vi "Constrained Nonlinear Optimization.vi"(0 "start":dbl[](array[numeric]), 1 "objective and constraint function":T3, 2 "function data":T2, 5 "bounds":T5, 9 "beginning state":T1, 11 "error in (no error)":errorcluster, 12 "cno settings":T6={"constraint weight"=1.0, "maximum minor iterations"=10}, 13 "stopping criteria":T4={"function tolerance"=1e-06, "parameter tolerance"=1e-06, "max iterations"=100, "max function calls"=1000, "gradient tolerance"=1e-06, "max time (sec)"=-1.0}) -> (3 "number of function calls":i32, 4 "minimum":dbl[](array[numeric]), 6 "f(minimum)":dbl, 10 "ending state":T1, 15 "error out":errorcluster)   [LabVIEW 2020, in "NI_Gmath.lvlib"]
doc: "Solves a general nonlinear optimization problem with nonlinear equality constraint and nonlinear inequality constraint bounds using a sequential quadratic programming method."
uses:
  NI_Gmath.lvlib
  cno_tuning parameters.ctl
  cno_bounds.ctl
  cno_initial values.ctl
  stopping criteria.ctl
  cno_user objective function ref.ctl
  objective function data.ctl
  NI_AALPro.lvlib
panel:
  in  "ending state 2":T1
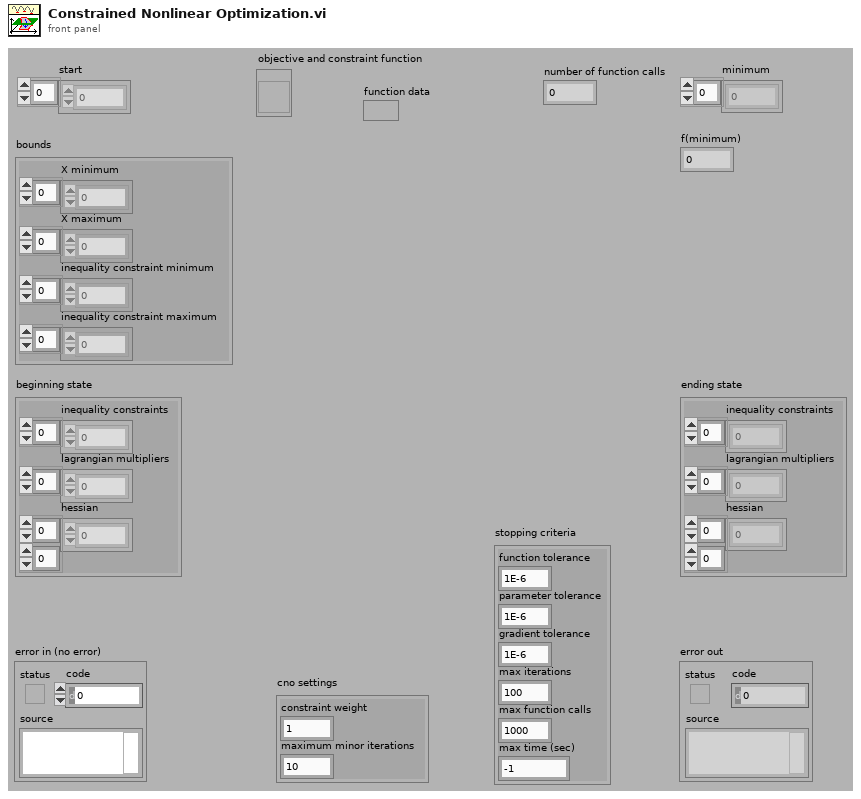
[diagram p1: front panel]
types:
  T1 = typedef "NI_Gmath.lvlib/cno_initial values.ctl" = cluster{"inequality constraints":dbl[], "lagrangian multipliers":dbl[], "hessian":dbl[][]}
  T2 = typedef "NI_Gmath.lvlib/objective function data.ctl" = variant
  T3 = typedef "NI_Gmath.lvlib/cno_user objective function ref.ctl" = refnum<vi>
  T4 = typedef "NI_Gmath.lvlib/stopping criteria.ctl" = cluster{"function tolerance":dbl, "parameter tolerance":dbl, "max iterations":i32, "max function calls":i32, "gradient tolerance":dbl, "max time (sec)":dbl}
  T5 = typedef "NI_Gmath.lvlib/cno_bounds.ctl" = cluster{"X minimum":dbl[], "X maximum":dbl[], "inequality constraint minimum":dbl[], "inequality constraint maximum":dbl[]}
  T6 = typedef "NI_Gmath.lvlib/cno_tuning parameters.ctl" = cluster{"constraint weight":dbl, "maximum minor iterations":i32}
  T7 = cluster{"objective and constraint function":T3, "function data":T2}
  T8 = typedef "NI_Gmath.lvlib/stopping criteria with time.ctl" = cluster{"function tolerance":dbl, "parameter tolerance":dbl, "max iterations":i32, "max function calls":i32, "gradient tolerance":dbl, "max time (sec)":dbl, "initial tick count":u32}
  T9 = typedef "NI_Gmath.lvlib/cno_data.ctl" = cluster{"NP":i32, "NIC":i32, "NEC":i32, "NC":i32, "NPIC":i32, "parameterBounds":bool, "alpha1":dbl, "alpha2":dbl, "alpha3":dbl, "alpha4":dbl, "CH":i32, "MM":i32, "tolerance":dbl}
  T10 = enum32{"Identity", "Diagonal", "Toepliz", "Vandermonde", "Companion"}
  T11 = typedef "NI_Matrix.lvlib/RealMatrix.ctl" = dbl[][]
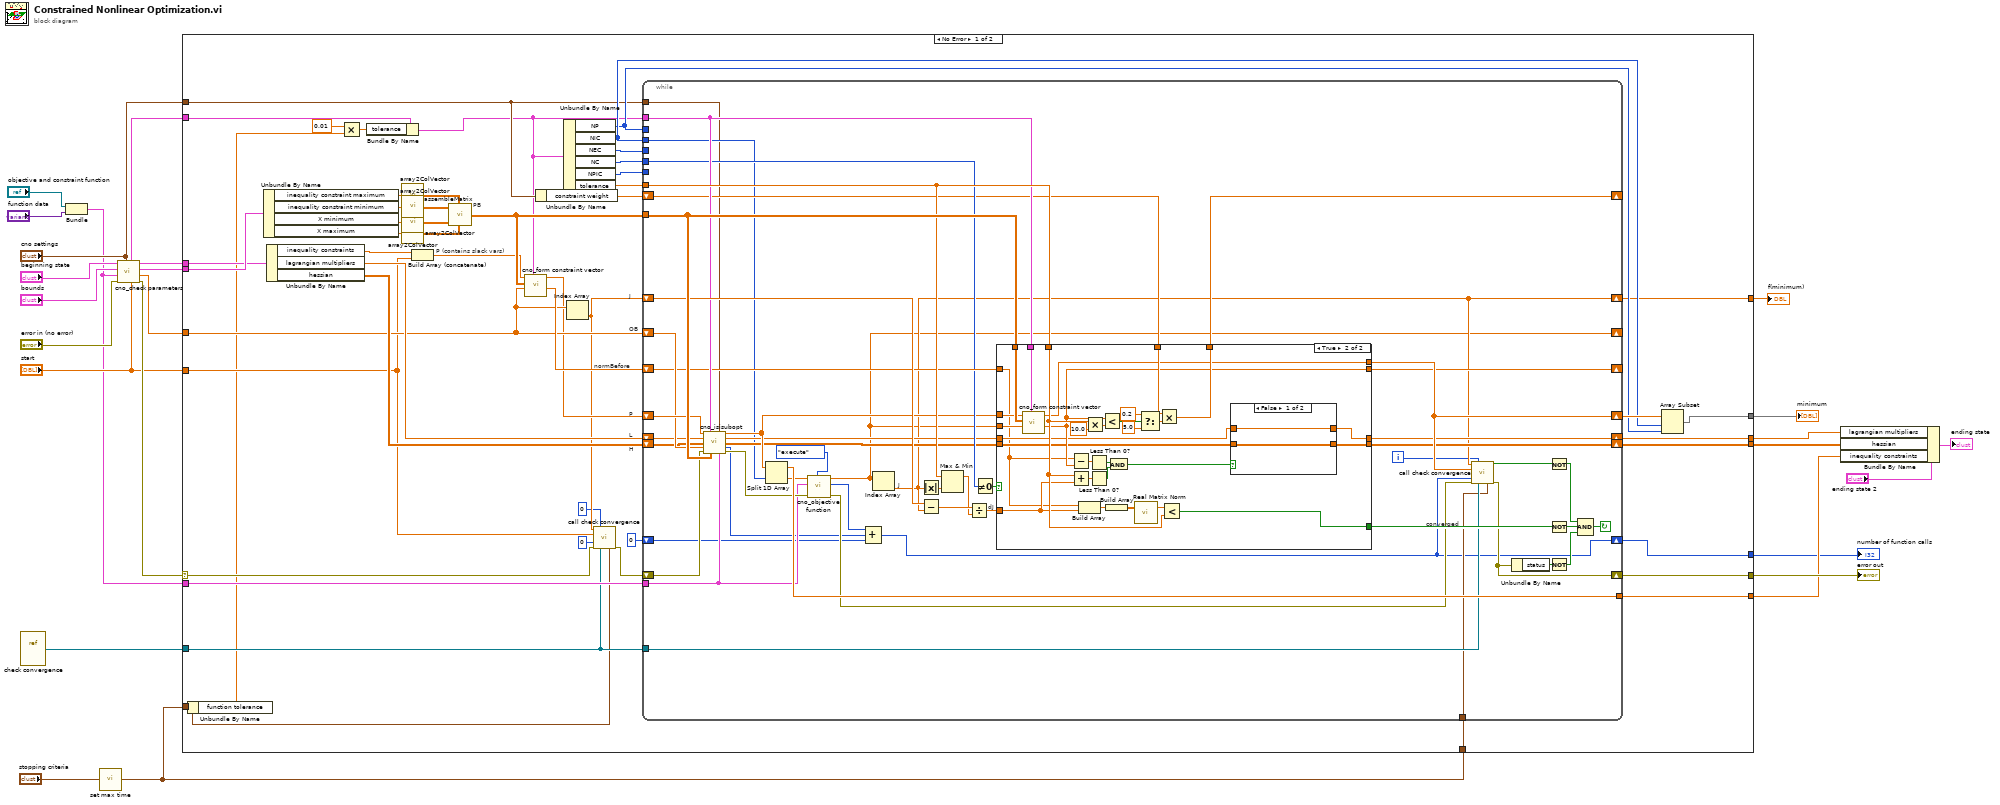
[diagram p0: block diagram]
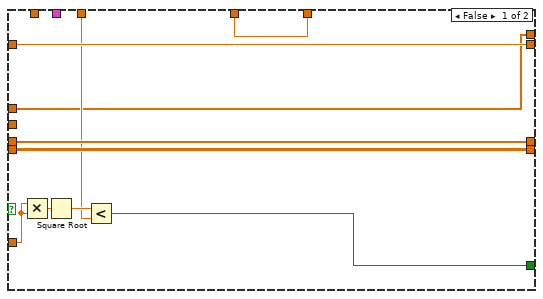
[diagram p2: hidden frame]
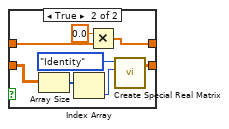
[diagram p3: hidden frame]
diagram:
  n1 = vi-ref "check convergence.vi"() -> ("vi reference"=w7:refnum<vi>)
  n2 = Bundle("objective and constraint function"="objective and constraint function", "function data"="function data") -> (w4:T7)  [unwired: 1 in]
  n3 = call "set max time.vi"("stopping criteria"="stopping criteria") -> ("stopping criteria"=w2:T8)
  n4 = call "cno_check parameters.vi"("initial parameters"="start", "tuning parameters"="cno settings", "error in (no error)"="error in (no error)", "user defined functions"=w4, "limits"="bounds", "state values"="beginning state") -> ("error out"=w19:errorcluster, "OB0"=w18:dbl[], "limits out"=w21:T5, "state values out"=w20:T1, "cno data"=w17:T9)  [unwired: 1 in]
  n5 = case shown="No Error" w19 {
    selector: w19 -> [w41 w176]
    tunnel: w4 -> [w58 _]
    tunnel: w20 -> [w74 _]
    tunnel: w21 -> [w75 _]
    tunnel: w18 -> [w56 _]
    tunnel: "cno settings" -> [w31 _]
    tunnel: w17 -> [w30 _]
    tunnel: [w55 w176] -> w16
    tunnel: [w49 _] -> w10
    tunnel: [w54 _] -> w13
    tunnel: [w53 _] -> w12
    tunnel: [w45 _] -> w15
    tunnel: [w52 _] -> w14
    tunnel: "start" -> [w43 _]
    tunnel: [w27 _] -> w8
    tunnel: w7 -> [w39 _]
    tunnel: w2 -> [w38 _]
    tunnel: w2 -> [w34 _]
    frame No Error {
      # "OB"
      # "H"
      # "L"
      # "P"
      # "normBefore"
      # "J"
      # "PB"
      # "P (contains slack vars)"
      n6 = Unbundle By Name(w34) -> ("function tolerance"=w33:dbl)
      n7 = Unbundle By Name(w75) -> ("inequality constraint maximum"=w44:dbl[], "inequality constraint minimum"=w70:dbl[], "X minimum"=w72:dbl[], "X maximum"=w71:dbl[])
      n8 = Unbundle By Name(w74) -> ("inequality constraints"=w73:dbl[], "lagrangian multipliers"=w62:dbl[], "hessian"=w61:dbl[][])
      n9 = Multiply(x=0.01, y=w33) -> (x*y=w32:dbl)
      n10 = Bundle By Name(cluster=w30, "tolerance"=w32) -> (w29:T9)
      n11 = call "array2ColVector.vi"("vector"=w44) -> ("col vector"=w66:dbl[][])
      n12 = call "array2ColVector.vi"("vector"=w70) -> ("col vector"=w67:dbl[][])
      n13 = call "array2ColVector.vi"("vector"=w72) -> ("col vector"=w69:dbl[][])
      n14 = call "array2ColVector.vi"("vector"=w71) -> ("col vector"=w68:dbl[][])
      n15 = Build Array (concatenate)(w73, w43) -> (w63:dbl[])
      n16 = call "assembleMatrix.vi"("A"=w67, "B"=w66, "C"=w69, "D"=w68) -> ("ABCD"=w65:dbl[][])  [unwired: 1 in]
      n17 = call "cno_form constraint vector.vi"("cno data"=w29, "OB"=w56, "PB"=w65, "P in"=w63) -> ("norm"=w64:dbl, "P out"=w51:dbl[])  [unwired: 6 in]
      n18 = Unbundle By Name(w31) -> ("constraint weight"=w57:dbl)
      n19 = Unbundle By Name(w29) -> ("NP"=w47:i32, "NIC"=w48:i32, "NEC"=w46:i32, "NC"=w60:i32, "NPIC"=w59:i32, "tolerance"=w28:dbl)
      n20 = Index Array(array=w56) -> (element=w42:dbl)  [unwired: 1 in]
      n21 = call "call check convergence.vi"("f"=w42, "current iteration"=0, "X"=w43, "number of function evaluations"=0, "error in"=w41, "vi reference"=w39, "stopping criteria"=w34) -> ("error out"=w40:errorcluster)  [unwired: 4 in, 4 out]
      n22 = while {
        tunnel: w65 -> [w124]
        shift-right: [w113] -> _
        shift-left: w64 -> [w109]
        tunnel: w31 -> [w86]
        shift-right: [w112] -> w52
        shift-left: w62 -> [w97]
        shift-right: [w111] -> w54
        shift-left: w61 -> [w99]
        shift-right: [w125] -> w50
        shift-left: w51 -> [w122]
        tunnel: w29 -> [w116]
        tunnel: w47 -> [_]
        tunnel: w48 -> [w95]
        tunnel: w46 -> [_]
        tunnel: w60 -> [w103]
        tunnel: w59 -> [_]
        shift-right: [w91] -> w55
        shift-left: w40 -> [w121]
        tunnel: w58 -> [w80]
        shift-right: [w94] -> w45
        shift-left: w42 -> [w120]
        tunnel: w28 -> [w123]
        shift-right: [w114] -> _
        shift-left: w57 -> [w100]
        shift-right: [w83] -> _
        shift-left: w56 -> [w115]
        tunnel: [w101] -> w53
        tunnel: w39 -> [w92]
        tunnel: w38 -> [w87]
        shift-right: [w76] -> w27
        shift-left: 0 -> [w78]
        i -> [w93]
        stop <- w88 continue-if-true
        # "J"
        # "converged"
        # "dJ"
        n23 = call "cno_isisubopt.vi"("P"=w122, "cno data"=w116, "tuning parameters"=w86, "L"=w97, "H"=w99, "OB"=w115, "error in (no error)"=w121, "PB"=w124, "user defined functions"=w80) -> ("P"=w102:dbl[], "L"=w96:dbl[], "H"=w98:dbl[][], "number of function calls"=w79:i32, "error out"=w82:errorcluster)  [unwired: 2 in]
        n24 = Split 1D Array(array=w102, index=w95) -> (first subarray=w101:dbl[], second subarray=w84:dbl[])
        n25 = call "cno_objective function.vi"("function"=enum16{"initialize", "execute"}."execute", "error in (no error)"=w82, "user defined functions"=w80, "X"=w84) -> ("error out"=w81:errorcluster, "num function calls"=w77:i32, "F(X)"=w83:dbl[])  [unwired: 5 in]
        n26 = Compound Arithmetic op=ADD(w77, w79, w78) -> (w76:i32)
        n27 = Index Array(array=w83) -> (element=w94:dbl)  [unwired: 1 in]
        n28 = Absolute Value(x=w94) -> (abs(x)=w119:dbl)
        n29 = Subtract(x=w120, y=w94) -> (x-y=w118:dbl)
        n30 = Max & Min(x=w123, y=w119) -> (max(x,y)=w117:dbl)  [unwired: 1 out]
        n31 = Divide(x=w118, y=w117) -> (x/y=w110:dbl)
        n32 = Not Equal To 0?(x=w103) -> (x != 0?=w104:bool)
        n33 = case shown="True" w104 {
          tunnel: w123 -> [w128 w165]
          tunnel: w124 -> [_ w164]
          tunnel: w116 -> [_ w163]
          tunnel: w102 -> [w126 w162]
          tunnel: w83 -> [_ w161]
          tunnel: w100 -> [w134 w154]
          tunnel: [w134 w153] -> w114
          tunnel: [w135 w152] -> w113
          tunnel: w98 -> [w132 w146]
          tunnel: w96 -> [w133 w145]
          tunnel: [w133 w144] -> w112
          tunnel: [w132 w143] -> w111
          tunnel: w110 -> [w131 w142]
          tunnel: w109 -> [w135 w141]
          tunnel: [w127 w139] -> w107
          tunnel: [w126 w138] -> w125
          frame False {
            n34 = Multiply(x=w131, y=w131) -> (x*y=w130:dbl)
            n35 = Square Root(x=w130) -> (sqrt(x)=w129:dbl)
            n36 = Less?(x=w129, y=w128) -> (x < y?=w127:bool)
          }
          frame True {
            n37 = call "cno_form constraint vector.vi"("cno data"=w163, "OB"=w161, "PB"=w164, "P in"=w162) -> ("norm"=w152:dbl, "P out"=w138:dbl[])  [unwired: 6 in]
            n38 = Subtract(x=w141, y=w152) -> (x-y=w151:dbl)
            n39 = Add(x=w165, y=w142) -> (x+y=w150:dbl)
            n40 = Build Array(w141, w142) -> (w137:dbl[])
            n41 = Multiply(x=w165, y=10.0) -> (x*y=w159:dbl)
            n42 = Less Than 0?(x=w151) -> (x < 0?=w149:bool)
            n43 = Less Than 0?(x=w150) -> (x < 0?=w148:bool)
            n44 = Less?(x=w152, y=w159) -> (x < y?=w158:bool)
            n45 = Build Array(w137) -> (w136:dbl[][])
            n46 = And(x=w149, y=w148) -> (x .and. y?=w147:bool)
            n47 = call "Real Matrix Norm.vi"("Input Matrix"=w136) -> ("norm"=w140:dbl)  [unwired: 1 in, 1 out]
            n48 = Select(t=0.2, s=w158, f=5.0) -> (s? t:f=w155:dbl)
            n49 = Multiply(x=w154, y=w155) -> (x*y=w153:dbl)
            n50 = Less?(x=w140, y=w165) -> (x < y?=w139:bool)
            n51 = case shown="False" w147 {
              tunnel: w146 -> [w166 w175]
              tunnel: w145 -> [w167 w170]
              tunnel: [w167 w168] -> w144
              tunnel: [w166 w171] -> w143
              frame False {
              }
              frame True {
                n52 = Array Size(array=w175) -> (size(s)=w174:i32[])
                n53 = Index Array(array=w174) -> (element=w173:i32)  [unwired: 1 in]
                n54 = Multiply(x=0.0, y=w170) -> (x*y=w168:dbl[])
                n55 = call "Create Special Real Matrix.vi"("matrix type"=T10."Identity", "matrix size"=w173) -> ("Special Matrix"=w171:T11)  [unwired: 3 in, 1 out]
              }
            }
          }
        }
        n56 = call "call check convergence.vi"("f"=w94, "current iteration"=w93, "X"=w125, "number of function evaluations"=w76, "error in"=w81, "vi reference"=w92, "stopping criteria"=w87) -> ("stop?"=w90:bool, "error out"=w91:errorcluster)  [unwired: 4 in, 3 out]
        n57 = Unbundle By Name(w91) -> ("status"=w106:bool)
        n58 = Not(x=w90) -> (.not. x?=w89:bool)
        n59 = Not(x=w107) -> (.not. x?=w108:bool)
        n60 = Not(x=w106) -> (.not. x?=w105:bool)
        n61 = Compound Arithmetic op=AND(w89, w108, w105) -> (w88:bool)
      }
      n62 = Array Subset(array=w50, index=w48, length=w47) -> (w49:dbl[])
    }
    frame Error {
    }
  }
  "f(minimum)" <- w15
  "error out" <- w16
  "minimum" <- w10
  "number of function calls" <- w8
  n63 = Bundle By Name(cluster="ending state 2", "lagrangian multipliers"=w14, "hessian"=w13, "inequality constraints"=w12) -> (→"ending state":T1)
